vi "Read Datalog File Example.vi"() -> ()   [LabVIEW 2011]
doc: "Opens the datalog file created by the Write Datalog File Example VI in this LLB and reads one record at a time from the file until all are read. Each record is a cluster containing a timestamp string and an array of single-precision numbers."
panel:
  in  "STOP":bool
  in  "NEXT RECORD":bool
  out "record data":sgl[](graph)
  out "record time":string
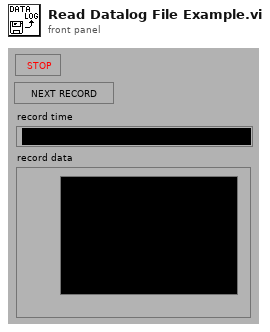
[diagram p1: front panel]
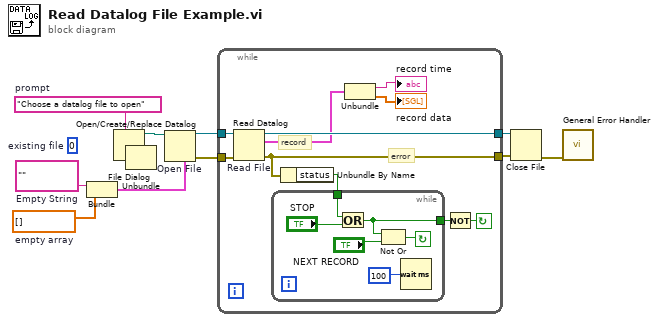
[diagram p0: block diagram]
diagram:
  (unwired) 0  # existing file
  w11 = sgl[] []  # empty array
  w10 = ""  # Empty String
  w6 = "Choose a datalog file to open"  # prompt
  n1 = Bundle(w10, "empty array"=w11) -> (w5:cluster{string, "empty array":sgl[]})  [unwired: 1 out]
  n2 = File Dialog(7:w6) -> (0:w1:errorcluster, 3:w7:path)  [unwired: 1 in, 7 out]
  n3 = Unbundle(w1) -> ()  [unwired: 3 out]
  n4 = Open/Create/Replace Datalog "Open File"(5:w5, 11:w7) -> (0:w8:errorcluster, 3:w9:refnum<k1>)  [unwired: 1 in, 4 out]
  n5 = while {
    tunnel: [w19] -> w4
    tunnel: w9 -> [w15]
    tunnel: [w18] -> w3
    tunnel: w8 -> [w16]
    stop <- w21 continue-if-true
    # "record"
    # "error"
    n6 = Read Datalog "Read File"(4:w16, 7:w15) -> (0:w18:errorcluster, 2:w14:cluster{string, "empty array":sgl[]}, 3:w19:refnum<k1>)  [unwired: 1 out]
    n7 = Unbundle By Name(w18) -> ("status"=w17:bool)
    n8 = while {
      tunnel: [w22] -> w20
      tunnel: w17 -> [w24]
      stop <- w26 continue-if-true
      n9 = Or(x=w24, y="STOP") -> (x .or. y?=w22:bool)
      n10 = Not Or(1:"NEXT RECORD", 2:w22) -> (0:w26:bool)
      n11 = Wait (ms)(milliseconds to wait=u32 100) -> ()  [unwired: 1 out]
    }
    n12 = Unbundle(w14) -> (→"record time":string, "empty array"=→"record data":sgl[])
    n13 = Not(x=w20) -> (.not. x?=w21:bool)
  }
  n14 = Close File(refnum=w4, error in=w3) -> (error out=w2:errorcluster)  [unwired: 1 out]
  n15 = call <vilib>:"General Error Handler.vi"("error in (no error)"=w2) -> ()  [unwired: 1 in, 14 out]
